vi "Testing Mode.vi"(8 "Filepath":path=path "D:/My Project/2019-2020/Magnetic Mareli UM/MM_UM/Project Setup/data/program seq/Program_280A.bin", 9 "FeedBack Channel":string[](array[string])=["fgdgfvcbc", "vnfhgjkn", "21354682"]) -> ()   [LabVIEW 2015]
uses:
  Control Button/Exit.ctl
  Control Button/Start.ctl
  Test  enqueue/AutoTest seq.ctl
  Control Button/Stop.ctl
  Control Button/Emergency.ctl
  Test  enqueue/Auot Test selection.ctl
  Galobal variable_TI.vi
  Project Setup/Globle Variable/GR_Servo.vi
  <vilib>/Utility/file.llb/Read Delimited Spreadsheet (string).vi
panel:
  out "Numeric":u32
  out "Error Message 2":string
  out "Sensor Setting Data":T1
  out "Sensor Data":T2
  out "Cllip-4 (AI12)":bool
  out "Cllip-3 (AI11)":bool
  out "Cllip-2(AI10)":bool
  out "Cllip-1 (AI9)":bool
  in  "Tracibility":bool=TRUE
  out "Home":bool
  out "Reset":bool
  out "Emergency":bool
  out "Start":bool
  out "Error   For Message":bool
  out "reset":bool
  out "D-enqueue":T3
  in  "Servo Fault Reset":bool
  out "Servo Fault":bool
  in  "Report":bool
  in  "Tab Control":enum32{"Test", "Report"}(tab)
  out "Error":bool
  out "User Name":string
  in  "Table Control":string[][](table)
  in  "OK Counter":string
  in  "NG Counter":string
  out "Running Model":string
  out "Date time":string
  out "TFT Barcode":string
  out "MIC Barcode":string
  out "2D Picture":picture
  out "Camera":bool
  out "Camera":bool
  out "Co-ordinate":string
  out "Test Name":string
  out "Error Message":string
  out "Boolean 2":bool
  in  "Report":i32(listbox)
  out "Key Pad AI1":bool
  out "Key Pad AI0":bool
  out "appended array":string[](array[string])
  in  "Sensor Feedback":T4(array[cluster])
  in  "Home Call":bool
  out "Start":bool
  in  "Cycle":i32
  in  "Slide Servo Home Call":bool
  in  "Emergency":T5
  in  "Stop":T6
  in  "Home Call":bool
  out "Current Date & Time":timestamp
  out "Cycle Time(Sec)":i32
  in  "Start":T7
  in  "Cycle Start Bit":bool
  in  "vi reference":refnum<vi>
  in  "Reset Ct.":bool
  out "error out":errorcluster
  in  "Tbl Refnum":refnum<vi>
  in  "Exit":T8
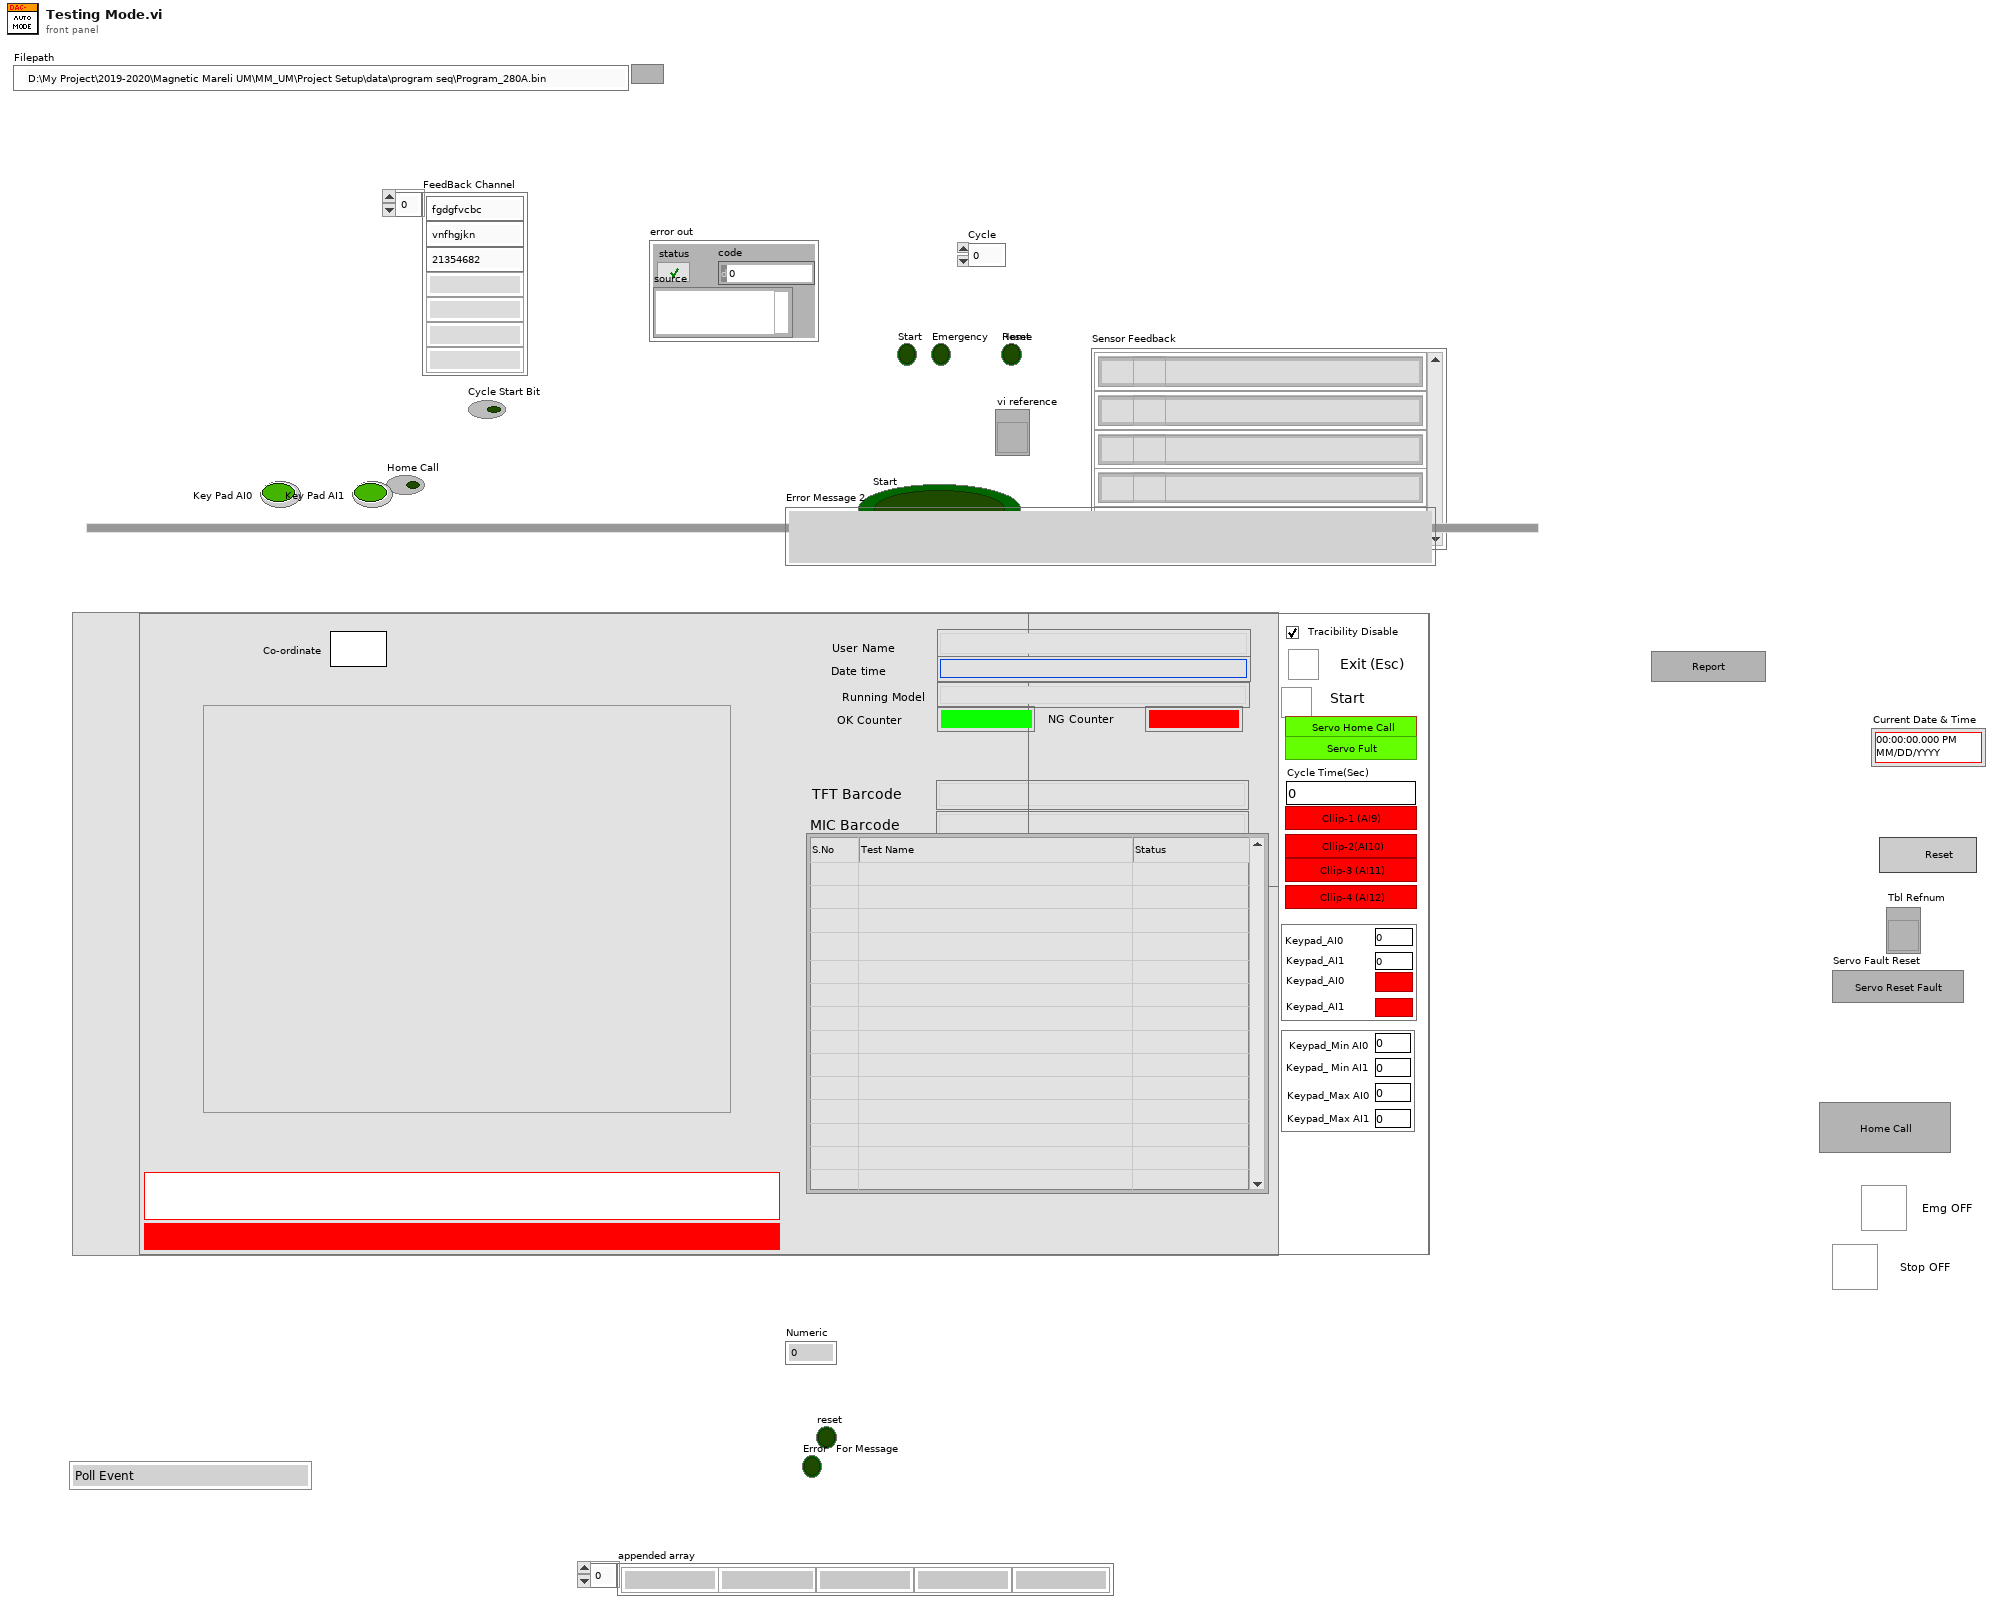
[diagram p1: front panel]
types:
  T1 = cluster{"Keypad_Max AI0":dbl, "Keypad_Min AI0":dbl, "Keypad_Max AI1":dbl, "Keypad_ Min AI1":dbl}
  T2 = cluster{"Keypad_AI0":dbl, "Keypad_AI1":dbl, "Keypad_AI0":bool, "Keypad_AI1":bool}
  T3 = typedef "AutoTest seq.ctl" = enum16{"Poll Event", "Part Clamp", "Program Seq", "Cylender Home", "Read Barcode", "Slide Servo send Cammand", "Slide Servo Home Call", "Camera Co-ordinate_1", "Camera Co-ordinate_2", "Result Save", "Error", "Exit"}
  T4 = cluster{"Sensor Name":string, "OK And NG":bool}[]
  T5 = typedef "Emergency.ctl" = bool
  T6 = typedef "Stop.ctl" = bool
  T7 = typedef "Start.ctl" = bool
  T8 = typedef "Exit.ctl" = bool
  T9 = cluster{"MIC ":refnum<visa-resource-name>, "baud rate MIC ":u32, "LCD ":refnum<visa-resource-name>, "baud rate_LCD":u32}
  T10 = typedef "Auot Test selection.ctl" = enum16{"Init", "Enqueue ", "Enqueue N", "Enqueue in stack", "Enqueue in stack N", "Dequeue", "Dequeue N", "Flush", "Release Queue"}
  T11 = cluster{"Item Name":string, "Item Status":bool, "Steps":cluster{"Channel Type":string, "Channels":string, "Wait/Poll (ms)":u32, "Parameter":u8, "STM-Speed":i32, "STM-Degree":u32, "Direction":u8}[]}[]
  T12 = enum16{"Part Clamp", "Part Unclamp", "Part Clamp Input Check", "Part Unclamp Input Check"}
  T13 = cluster{"No. Fail Coun t":string, "Rework Status Count 0\\1":string, "NA Count Max =3 ":string, "Testesd Count  0/1":string, "Error code":string}
  T14 = cluster{"Emergency_1":bool, "Reset_2":bool, "Air Pressure_4":bool, "Safety Sensor_5":bool, "Safety Sensor_6":bool, "Barcode Rev rs_24":bool, "Clamp fwd rs_21":bool, "Servo Fault":bool, "Home _3":bool}
  T15 = cluster{"IL Sensor1_Max AI0":dbl, "IL Sensor1_Min AI0":dbl, "IL Sensor1_Max AI1":dbl, "IL Sensor1_ Min AI1":dbl, "IL Sensor_Max (AI9)":dbl, "IL Sensor_Min  (AI9)":dbl, "IL Sensor_Max (AI10)":dbl, "IL Sensor_Min(AI10)":dbl, "IL Sensor_Max (AI11)":dbl, "IL Sensor_Min (AI11)":dbl, "IL Sensor_Max (AI12)":dbl, "IL Sensor_Min (AI12":dbl}
  T16 = cluster{"IL Sensor1_AI0":dbl, "IL Sensor1_AI1":dbl, "IL Sensor (AI6)":dbl, "IL Sensor  (AI7)":dbl, "IL Sensor (AI8)":dbl, "IL Sensor  (AI9)":dbl, "IL Sensor1_AI0":bool, "IL Sensor1_AI1":bool, "IL Sensor1_AI9":bool, "IL Sensor1_AI10":bool, "IL Sensor1_AI11":bool, "IL Sensor1_AI12":bool}
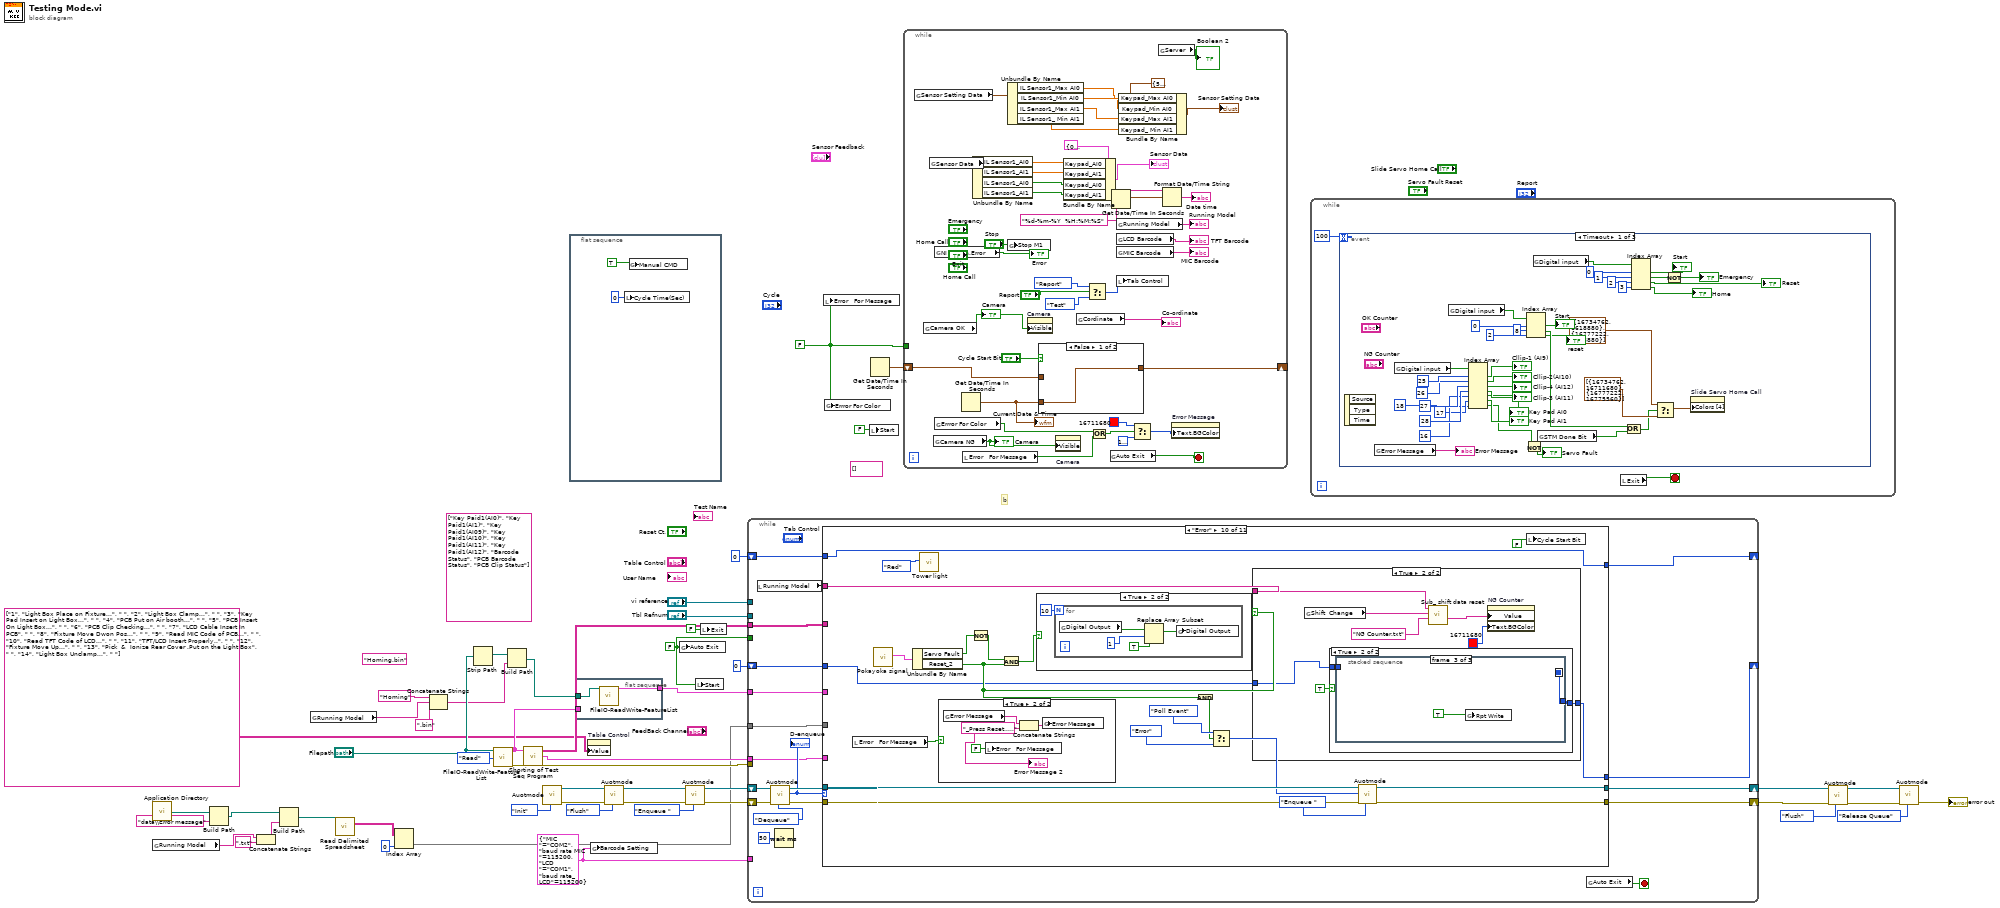
[diagram p0: block diagram]
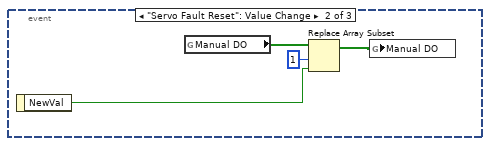
[diagram p2: hidden frame]
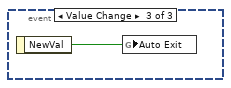
[diagram p3: hidden frame]
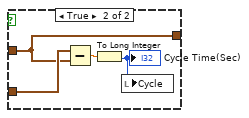
[diagram p4: hidden frame]
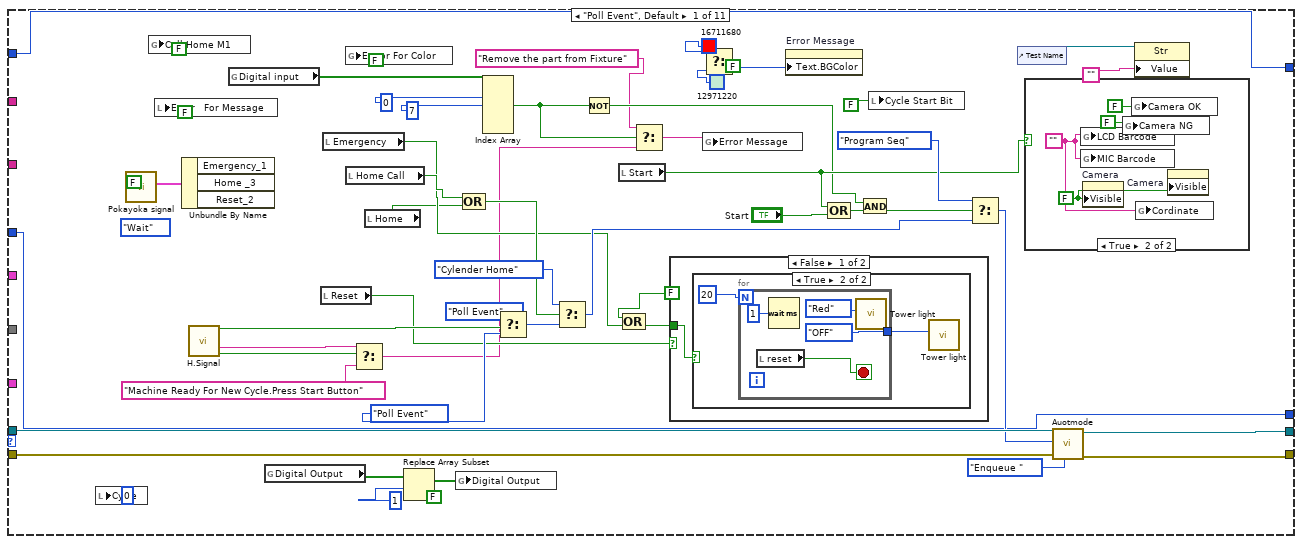
[diagram p5: hidden frame]
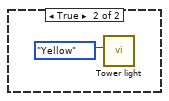
[diagram p8: hidden frame]
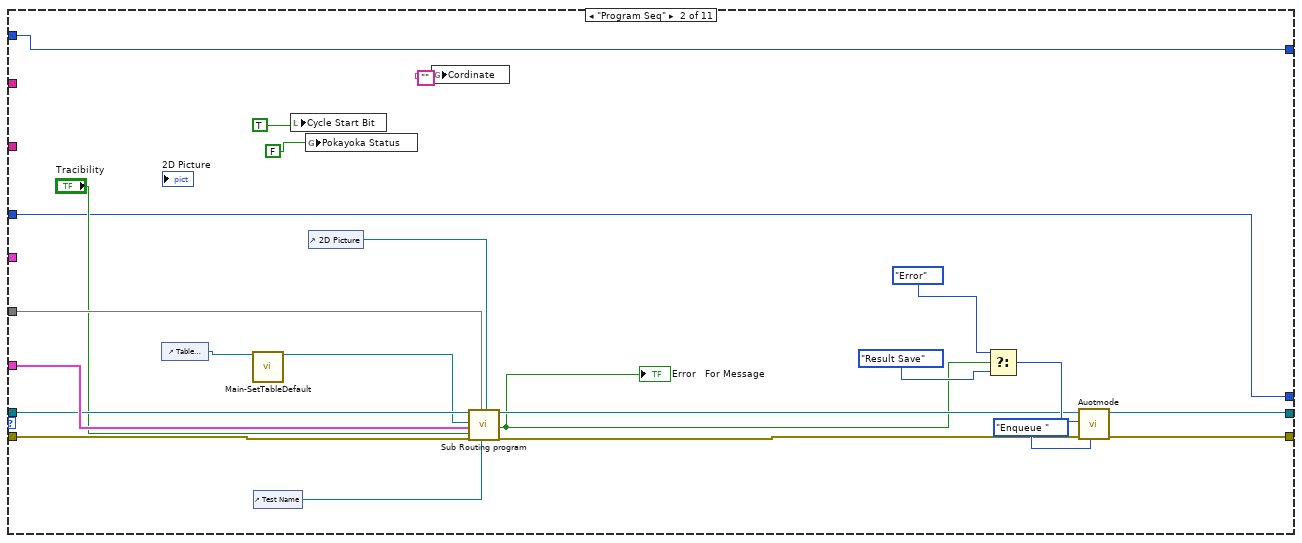
[diagram p9: hidden frame]
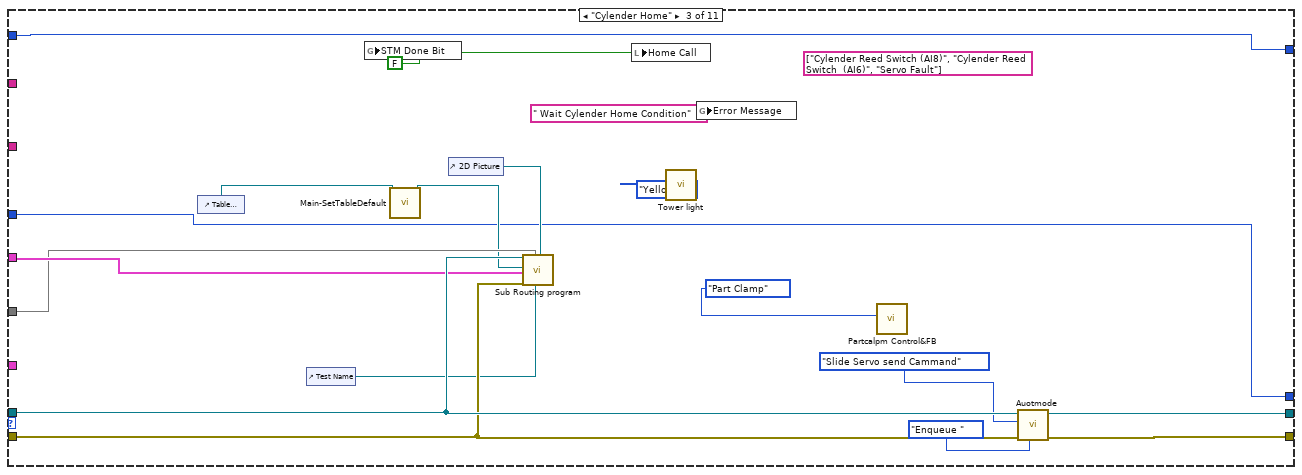
[diagram p10: hidden frame]
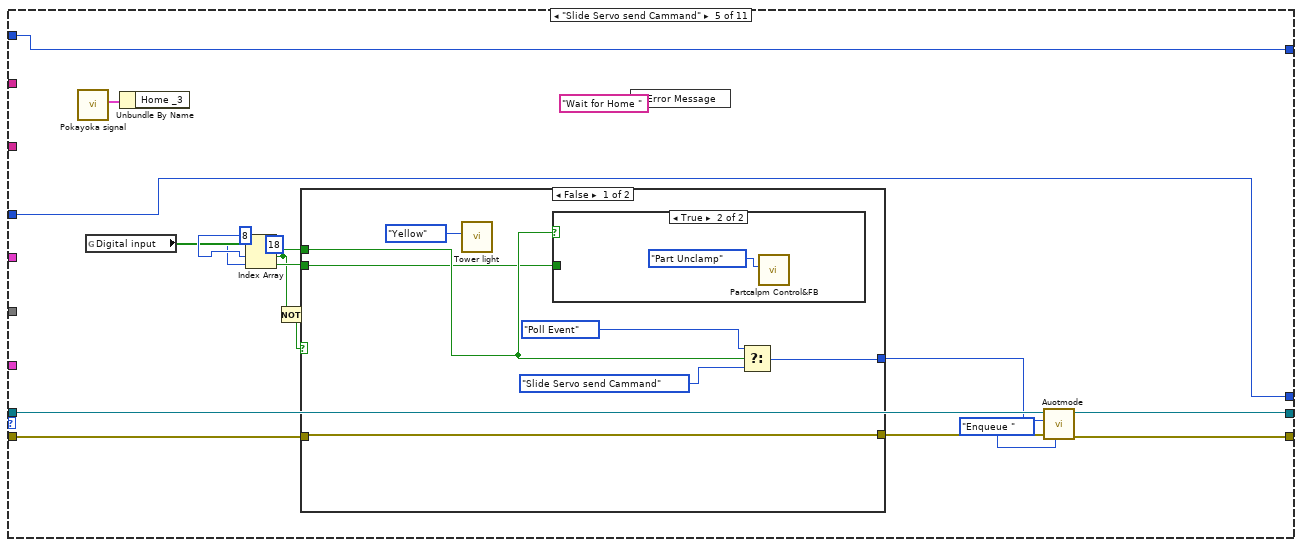
[diagram p12: hidden frame]
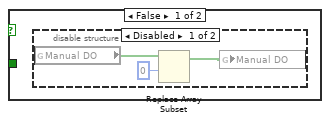
[diagram p13: hidden frame]
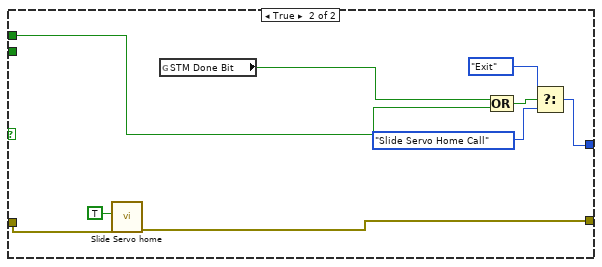
[diagram p15: hidden frame]
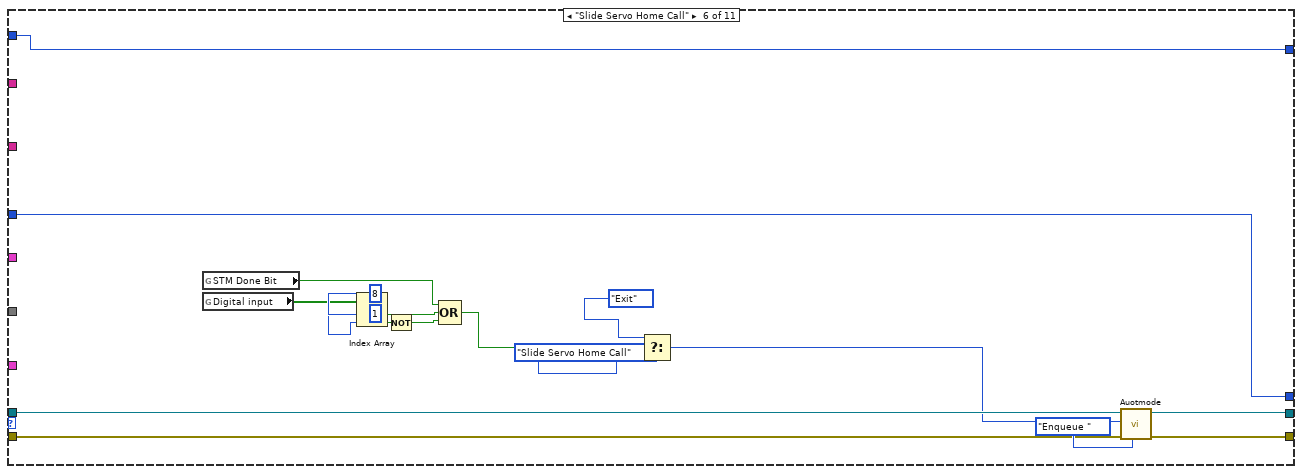
[diagram p16: hidden frame]
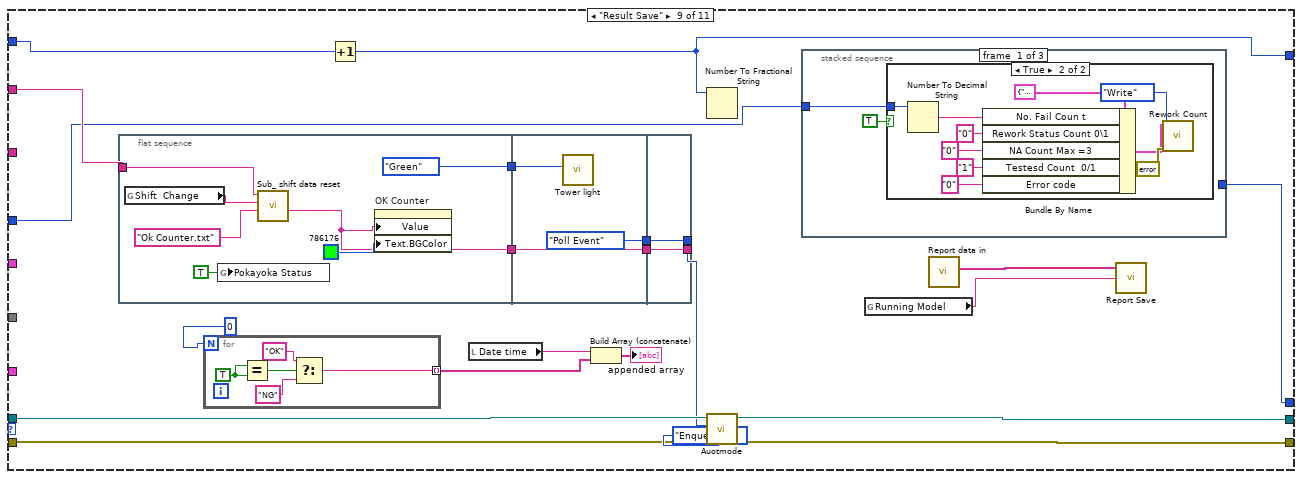
[diagram p19: hidden frame]
diagram:
  w20 = T9 {"MIC "="COM2", "baud rate MIC "=115200, "LCD "="COM1", "baud rate_LCD"=115200} ("Barcode Setting")
  (unwired) "Homing.bin" ("name or relative path")
  (unwired) string[] ["Key Paid1(AI0)", "Key Paid1(AI1)", "Key Paid1(AI09)", "Key Paid1(AI10)", "Key Paid1(AI11)", "Key Paid1(AI12)", "Barcode Status", "PCB Barcode Status", "PCB Clip Status"] ("Error Name")
  (unwired) string[] []
  w4 = FALSE ("Servo Stop")
  w27 = FALSE ("Auto Exit")
  # "b"
  n1 = call <vilib>:"Application Directory.vi"() -> ("Application Directory"=w14:path)
  n2 = global read "Galobal variable_TI.vi" "Running Model"() -> (w11:string)
  n3 = Build Path(base path=w14, name or relative path="data\\Error message") -> (appended path=w12:path)
  n4 = Concatenate Strings(w11, ".txt" ("string")) -> (w9:string)
  n5 = Build Path(base path=w12, name or relative path=w9) -> (appended path=w8:path)
  n6 = global read "Galobal variable_TI.vi" "Running Model"() -> (w18:string)
  n7 = call-poly <vilib>:"Read Delimited Spreadsheet.vi"("file path (dialog if empty)"=w8) -> ("all rows"=w7:string[][])  [unwired: 9 in, 5 out]
  n8 = Index Array(array=w7, index (col)=0 ("disabled index (col)")) -> (element=w5:string[])  [unwired: 1 in]
  n9 = Concatenate Strings("Homing" ("string"), w18, ".bin" ("string")) -> (w16:string)
  n10 = Strip Path(path="Filepath") -> (stripped path=w24:path)  [unwired: 1 out]
  n11 = call "FileIO-ReadWrite-FeatureList.vi"("Filepath"="Filepath", "Read/Write"=enum16{"Read", "Write"}."Read") -> ("Feature List (Out)"=w22:T11, "Error Out"=w32:errorcluster)  [unwired: 12 in]
  n12 = Build Path(base path=w24, name or relative path=w16) -> (appended path=w23:path)
  n13 = call "Shorting of Test Seq Program.vi"("Feature List (Out)"=w22) -> ("Feature Step Enable"=w28:T11, "Feature Name"=w3:string[][])  [unwired: 3 in]
  n14 = call "Auotmode.vi"("Enum Selection"=Auot_Test_selection."Init") -> ("error out"=w44:errorcluster, "queue Out"=w42:refnum<queue>)  [unwired: 7 in, 1 out]
  n15 = flat-sequence {
    frame #0 {
      n16 = local write "Cycle Time(Sec)"(0 ("Cycle Time(Sec)")) -> ()
      n17 = global write "Galobal variable_TI.vi" "Manual CMD"(TRUE ("Manual CMD")) -> ()
    }
  }
  n18 = flat-sequence {
    tunnel: w23 -> [w54]
    tunnel: w22 -> [_]
    tunnel: [w53] -> w21
    frame #0 {
      n19 = call "FileIO-ReadWrite-FeatureList.vi"("Filepath"=w54) -> ("Feature List (Out)"=w53:T11)  [unwired: 13 in, 1 out]
    }
  }
  n20 = property on="Table Control" class="Tbl (strict)"("Value"=string[][] [["1", "Light Box Place on Fixture...", " "], ["2", "Light Box Clamp...", " "], ["3", "Key Pad Insert on Light Box...", " "], ["4", "PCB Put on Air booth...", " "], ["5", "PCB Insert On Light Box...", " "], ["6", "PCB Clip Checking...", " "], ["7", "LCD Cable Insert In PCB", " "], ["8", "Fixture Move Dwon Pos...", " "], ["9", "Read MIC Code of PCB...", " "], ["10", "Read TFT Code of LCD...", " "], ["11", "TFT/LCD Insert Properly..", " "], ["12", "Fixture Move Up...", " "], ["13", "Pick  &  Ionize Rear Cover .Put on the Light Box", " "], ["14", "Light Box Unclamp...", " "]] ("Table Control 2")) -> ()  [unwired: 2 in, 2 out]
  n21 = global write "Galobal variable_TI.vi" "Barcode Setting"(w20) -> ()
  n22 = call "Auotmode.vi"("Enum Selection"=Auot_Test_selection."Flush", "Error In"=w44, "queue in"=w42) -> ("error out"=w43:errorcluster, "queue Out"=w41:refnum<queue>)  [unwired: 5 in, 1 out]
  n23 = global write "Galobal variable_TI.vi" "Auto Exit"(w27) -> ()
  n24 = call "Auotmode.vi"("Enum Selection"=Auot_Test_selection."Enqueue ", "Error In"=w43, "queue in"=w41) -> ("error out"=w48:errorcluster, "queue Out"=w30:refnum<queue>)  [unwired: 5 in, 1 out]
  n25 = local write "Start"(w27) -> ()
  n26 = local write "Exit"(T8 FALSE ("Exit")) -> ()
  n27 = while {
    tunnel: "vi reference" -> [_]
    tunnel: "Tbl Refnum" -> [_]
    tunnel: w28 -> [w66]
    tunnel: w32 -> [_]
    tunnel: w5 -> [w67]
    shift-right: [w70] -> w35
    shift-left: w30 -> [w63]
    shift-right: [w62] -> w29
    shift-left: w48 -> [w72]
    tunnel: w27 -> [_]
    tunnel: w3 -> [w61]
    tunnel: w21 -> [w59]
    tunnel: w20 -> [_]
    shift-right: [w57] -> _
    shift-left: u32 0 ("milliseconds to wait") -> [w58]
    shift-right: [w55] -> _
    shift-left: u32 0 ("milliseconds to wait") -> [w56]
    stop <- w65 stop-if-true
    n28 = local read "Running Model"() -> (w60:string)
    n29 = call "Auotmode.vi"("Enum Selection"=Auot_Test_selection."Dequeue", "Error In"=w72, "queue in"=w63) -> ("error out"=w69:errorcluster, "D-enqueue"=w68:T3, "queue Out"=w71:refnum<queue>)  [unwired: 5 in]
    "D-enqueue" <- w68
    n30 = Wait (ms)(milliseconds to wait=u32 50) -> ()  [unwired: 1 out]
    n31 = case shown="\"Error\"" w68 {
      tunnel: w71 -> [w126 w151 w175 w183 w195 w235 w242 w246 w266 w319 w365]
      tunnel: [w124 w157 w178 w183 w199 w236 w242 w246 w264 w318 w366] -> w70
      tunnel: w69 -> [w125 w153 w174 w182 w197 w234 w241 w245 w265 w317 w367]
      tunnel: [w123 w156 w177 w182 w198 w237 w241 w245 w263 w316 w367] -> w62
      tunnel: w66 -> [_ w154 _ _ _ _ _ _ _ _ _]
      tunnel: w67 -> [_ w155 w172 _ _ _ _ _ _ _ _]
      tunnel: w61 -> [_ _ _ _ _ _ _ _ _ _ _]
      tunnel: w60 -> [_ _ _ _ _ _ _ _ w262 w310 _]
      tunnel: w59 -> [_ _ w173 _ _ _ _ _ _ _ _]
      tunnel: w58 -> [w87 w142 w163 w181 w185 w222 w240 w244 w251 w302 w358]
      tunnel: [w87 w142 w163 w181 w185 w222 w240 w244 w250 w302 w358] -> w57
      tunnel: w56 -> [w80 w139 w162 w180 w184 w221 w239 w243 w248 w301 w357]
      tunnel: [w80 w139 w162 w180 w184 w221 w239 w243 w247 w300 w357] -> w55
      frame "Poll Event", Default {
        (unwired) enum16{"Wait", "Ionizer On", "Ionizer off"}."Wait" ("Enum")
        (unwired) FALSE ("Ionizer cnf")
        n32 = local write "Cycle"(0 ("Cycle")) -> ()
        n33 = call "Pokayoka signal.vi"() -> ("output cluster"=w105:T14)  [unwired: 10 in, 1 out]
        n34 = global write "Galobal variable_TI.vi" "Call Home M1"(FALSE ("Call Home M1")) -> ()
        n35 = local write "Error   For Message"(FALSE ("Error   For Message")) -> ()
        n36 = Unbundle By Name(w105) -> ()  [unwired: 3 out]
        n37 = call "H.Signal.vi"() -> ("Slide servo home RS"=w111:bool, "Error Message"=w112:string, "Bool_H Sig"=w99:bool)  [unwired: 10 in, 3 out]
        n38 = global read "Galobal variable_TI.vi" "Digital input"() -> (w121:bool[])
        n39 = global read "Galobal variable_TI.vi" "Digital Output"() -> (w96:bool[])
        n40 = local read "Reset"() -> (w83:bool)
        n41 = local read "Emergency"() -> (w85:bool)
        n42 = global write "Galobal variable_TI.vi" "Errror For Color"(FALSE ("Errror For Color")) -> ()
        n43 = local read "Home Call"() -> (w97:bool)
        n44 = Select(t=w112, s=w99, f="Machine Ready For New Cycle.Press Start Button") -> (s? t:f=w74:string)
        n45 = local read "Home"() -> (w84:bool)
        n46 = Replace Array Subset(array=w96, new element=FALSE ("new element/subarray"), index=1) -> (w95:bool[])
        n47 = global write "Galobal variable_TI.vi" "Digital Output"(w95) -> ()
        n48 = Compound Arithmetic op=OR(w97, w84) -> (w118:bool)
        n49 = Index Array(array=w121, index #1=0 ("index"), index #2=7 ("index")) -> (element #2=w75:bool)  [unwired: 3 in, 4 out]
        n50 = Select(t=AutoTest_seq."Poll Event" ("Enqueue"), s=w111, f=AutoTest_seq."Poll Event") -> (s? t:f=w116:T3)
        n51 = Select(t=AutoTest_seq."Cylender Home" ("Enqueue"), s=w118, f=w116) -> (s? t:f=w104:T3)
        n52 = Not(x=w75) -> (.not. x?=w78:bool)
        n53 = local read "Start"() -> (w86:bool)
        n54 = Compound Arithmetic op=OR(FALSE ("value"), w85) -> (w100:bool)
        n55 = Select(t="Remove the part from Fixture", s=w75, f=w74) -> (s? t:f=w77:string)
        n56 = case shown="False" w83 {
          tunnel: w100 -> [w131 _]
          frame False {
            n57 = case shown="True" w131 {
              frame False {
              }
              frame True {
                n58 = for {
                  N: 20 -> [_]
                  tunnel: [enum16{"Green", "Red", "Yellow", "OFF"}."OFF" ("Enum")] -> w132
                  stop <- w134 stop-if-true
                  n59 = local read "reset"() -> (w134:bool)
                  n60 = Wait (ms)(milliseconds to wait=u32 1) -> ()  [unwired: 1 out]
                  n61 = call "Tower light.vi"("Enum"=enum16{"Green", "Red", "Yellow"}."Red") -> ()  [unwired: 11 in]
                }
                n62 = call "Tower light.vi"("Enum"=w132) -> ()  [unwired: 11 in]
              }
            }
          }
          frame True {
            n63 = call "Tower light.vi"("Enum"=enum16{"Green", "Red", "Yellow"}."Yellow") -> ()  [unwired: 11 in]
          }
        }
        n64 = global write "GR_Servo.vi" "Error Message"(w77) -> ()
        n65 = Select(t=u32 16711680, s=FALSE, f=u32 12971220) -> (s? t:f=w88:u32)
        n66 = property on="Error Message" class="Str"("Text.BGColor"=w88) -> ()  [unwired: 2 in, 2 out]
        n67 = Compound Arithmetic op=OR(w86, "Start") -> (w109:T7)
        n68 = And(x=w78, y=w109) -> (x .and. y?=w79:T7)
        n69 = local write "Cycle Start Bit"(FALSE ("Cycle Start Bit")) -> ()
        n70 = Select(t=AutoTest_seq."Program Seq" ("Enqueue"), s=w79, f=w104) -> (s? t:f=w103:T3)
        n71 = control-ref of="Test Name"() -> (w102:refnum<vi>)
        n72 = case shown="True" w86 {
          frame False {
          }
          frame True {
            w130 = FALSE ("Visible")
            w127 = ""
            n73 = global write "Galobal variable_TI.vi" "LCD Barcode"(w127) -> ()
            n74 = global write "Galobal variable_TI.vi" "MIC Barcode"(w127) -> ()
            n75 = property on="Camera" class="Bool (strict)"("Visible"=w130) -> ()  [unwired: 2 in, 2 out]
            n76 = global write "Galobal variable_TI.vi" "Camera NG"(FALSE ("Camera NG")) -> ()
            n77 = global write "Galobal variable_TI.vi" "Camera OK"(FALSE ("Camera OK")) -> ()
            n78 = global write "Galobal variable_TI.vi" "Cordinate"(w127) -> ()
            n79 = property on="Camera" class="Bool (strict)"("Visible"=w130) -> ()  [unwired: 2 in, 2 out]
          }
        }
        n80 = call "Auotmode.vi"("Enum Selection"=Auot_Test_selection."Enqueue ", "Error In"=w125, "Enqueue"=w103, "queue in"=w126) -> ("error out"=w123:errorcluster, "queue Out"=w124:refnum<queue>)  [unwired: 4 in, 1 out]
        n81 = property class="Str"(reference=w102, "Value"="") -> ()  [unwired: 1 in, 2 out]
      }
      frame "Program Seq" {
        n82 = control-ref of="Table Control"() -> (w147:refnum<vi>)
        n83 = call "Main-SetTableDefault.vi"("Table (In)"=w147) -> ("Table (Out)"=w146:refnum<vi>)  [unwired: 13 in, 1 out]
        n84 = control-ref of="Test Name"() -> (w149:refnum<vi>)
        n85 = local write "Cycle Start Bit"(TRUE ("Cycle Start Bit")) -> ()
        n86 = global write "Galobal variable_TI.vi" "Pokayoka Status"(FALSE ("Pokayoka Status")) -> ()
        n87 = control-ref of="2D Picture"() -> (w148:refnum<vi>)
        n88 = global write "Galobal variable_TI.vi" "Cordinate"("") -> ()
        n89 = call "Sub Routing program.vi"("queue Out in"=w151, "Table"=w146, "Feature Step Enable"=w154, "error in (no error)"=w153, "Tracibility"="Tracibility", "FeedBack Channel"=w155, "Test Name"=w149, "Image"=w148) -> ("Queue out"=w150:refnum<queue>, "Error"=w143:bool, "error out"=w152:errorcluster)  [unwired: 8 in, 1 out]
        "Error   For Message" <- w143
        n90 = Select(t=AutoTest_seq."Error" ("Enqueue"), s=w143, f=AutoTest_seq."Result Save" ("Enqueue")) -> (s? t:f=w158:T3)
        n91 = call "Auotmode.vi"("Enum Selection"=Auot_Test_selection."Enqueue ", "Error In"=w152, "Enqueue"=w158, "queue in"=w150) -> ("error out"=w156:errorcluster, "queue Out"=w157:refnum<queue>)  [unwired: 4 in, 1 out]
      }
      frame "Cylender Home" {
        (unwired) string[] ["Cylender Reed Switch (AI8)", "Cylender Reed Switch  (AI6)", "Servo Fault"]
        w176 = FALSE ("STM Done Bit")
        n92 = control-ref of="Table Control"() -> (w168:refnum<vi>)
        n93 = control-ref of="Test Name"() -> (w171:refnum<vi>)
        n94 = global write "Galobal variable_TI.vi" "STM Done Bit"(w176) -> ()
        n95 = call "Main-SetTableDefault.vi"("Table (In)"=w168) -> ("Table (Out)"=w167:refnum<vi>)  [unwired: 13 in, 1 out]
        n96 = control-ref of="2D Picture"() -> (w170:refnum<vi>)
        n97 = call "Sub Routing program.vi"("queue Out in"=w175, "Table"=w167, "Feature Step Enable"=w173, "error in (no error)"=w174, "FeedBack Channel"=w172, "Test Name"=w171, "Image"=w170) -> ()  [unwired: 9 in, 4 out]
        n98 = local write "Home Call"(w176) -> ()
        n99 = call "Tower light.vi"("Enum"=enum16{"Green", "Red", "Yellow"}."Yellow") -> ()  [unwired: 11 in]
        n100 = global write "GR_Servo.vi" "Error Message"(" Wait Cylender Home Condition") -> ()
        n101 = call "Partcalpm Control&FB.vi"("Enum"=T12."Part Clamp") -> ()  [unwired: 9 in, 2 out]
        n102 = call "Auotmode.vi"("Enum Selection"=Auot_Test_selection."Enqueue ", "Error In"=w174, "Enqueue"=AutoTest_seq."Slide Servo send Cammand", "queue in"=w175) -> ("error out"=w177:errorcluster, "queue Out"=w178:refnum<queue>)  [unwired: 4 in, 1 out]
      }
      frame "Read Barcode" {
      }
      frame "Slide Servo send Cammand" {
        n103 = call "Pokayoka signal.vi"() -> ("output cluster"=w193:T14)  [unwired: 10 in, 1 out]
        n104 = global read "Galobal variable_TI.vi" "Digital input"() -> (w190:bool[])
        n105 = Unbundle By Name(w193) -> ()  [unwired: 1 out]
        n106 = Index Array(array=w190, index #1=8 ("index"), index #2=18 ("index")) -> (element #1=w187:bool, element #2=w188:bool)
        n107 = Not(x=w187) -> (.not. x?=w186:bool)
        n108 = case shown="False" w186 {
          tunnel: w197 -> [w207 w220]
          tunnel: [w207 w219] -> w196
          tunnel: [w203 w214] -> w194
          tunnel: w187 -> [w202 w212]
          tunnel: w188 -> [w201 _]
          frame False {
            n109 = call "Tower light.vi"("Enum"=enum16{"Green", "Red", "Yellow"}."Yellow") -> ()  [unwired: 11 in]
            n110 = case shown="True" w202 {
              tunnel: w201 -> [_ _]
              frame False {
                n111 = disable-structure shown="Disabled" {
                  frame Disabled {
                    n112 = global read "Galobal variable_TI.vi" "Manual DO"() -> (w210:bool[])
                    n113 = Replace Array Subset(array=w210, index=0) -> (w209:bool[])  [unwired: 1 in]
                    n114 = global write "Galobal variable_TI.vi" "Manual DO"(w209) -> ()
                  }
                  frame Enabled {
                  }
                }
              }
              frame True {
                n115 = call "Partcalpm Control&FB.vi"("Enum"=T12."Part Unclamp") -> ()  [unwired: 9 in, 2 out]
              }
            }
            n116 = Select(t=AutoTest_seq."Poll Event" ("Enqueue"), s=w202, f=AutoTest_seq."Slide Servo send Cammand" ("Enqueue")) -> (s? t:f=w203:T3)
          }
          frame True {
            n117 = call "Slide Servo home.vi"("error in"=w220, "NewVal"=TRUE) -> ("error out"=w219:errorcluster)  [unwired: 9 in]
            n118 = global read "Galobal variable_TI.vi" "STM Done Bit"() -> (w217:bool)
            n119 = Compound Arithmetic op=OR(w217, w212) -> (w213:bool)
            n120 = Select(t=AutoTest_seq."Exit" ("Enqueue"), s=w213, f=AutoTest_seq."Slide Servo Home Call" ("Enqueue")) -> (s? t:f=w214:T3)
          }
        }
        n121 = global write "GR_Servo.vi" "Error Message"("Wait for Home ") -> ()
        n122 = call "Auotmode.vi"("Enum Selection"=Auot_Test_selection."Enqueue ", "Error In"=w196, "Enqueue"=w194, "queue in"=w195) -> ("error out"=w198:errorcluster, "queue Out"=w199:refnum<queue>)  [unwired: 4 in, 1 out]
      }
      frame "Slide Servo Home Call" {
        n123 = global read "Galobal variable_TI.vi" "STM Done Bit"() -> (w228:bool)
        n124 = global read "Galobal variable_TI.vi" "Digital input"() -> (w226:bool[])
        n125 = Index Array(array=w226, index #1=8 ("index"), index #2=1 ("index")) -> (element #1=w227:bool, element #2=w224:bool)
        n126 = Not(x=w224) -> (.not. x?=w223:bool)
        n127 = Compound Arithmetic op=OR(w228, w227, w223) -> (w230:bool)
        n128 = Select(t=AutoTest_seq."Exit" ("Enqueue"), s=w230, f=AutoTest_seq."Slide Servo Home Call" ("Enqueue")) -> (s? t:f=w233:T3)
        n129 = call "Auotmode.vi"("Enum Selection"=Auot_Test_selection."Enqueue ", "Error In"=w234, "Enqueue"=w233, "queue in"=w235) -> ("error out"=w237:errorcluster, "queue Out"=w236:refnum<queue>)  [unwired: 4 in, 1 out]
      }
      frame "Camera Co-ordinate_1" {
      }
      frame "Camera Co-ordinate_2" {
      }
      frame "Result Save" {
        n130 = flat-sequence {
          tunnel: w262 -> [w292]
          tunnel: [enum16{"Green", "Red", "Yellow"}."Green" ("Enum")] -> w261
          tunnel: [w289] -> w253
          tunnel: w261 -> [w297]
          tunnel: [AutoTest_seq."Poll Event" ("Enqueue")] -> w259
          tunnel: [w295] -> w254
          tunnel: w253 -> [w295]
          tunnel: [w299] -> w260
          tunnel: w259 -> [w299]
          tunnel: [w298] -> _
          tunnel: w254 -> [w298]
          frame #0 {
            n131 = global read "Galobal variable_TI.vi" "Shift  Change"() -> (w288:string)
            n132 = global write "Galobal variable_TI.vi" "Pokayoka Status"(TRUE ("Pokayoka Status")) -> ()
            n133 = call "Sub_ shift data reset.vi"("Serial no"="Ok Counter.txt" ("File Name"), "Shift"=w288, "Model"=w292) -> ("Serial no"=w289:string)  [unwired: 6 in, 1 out]
            n134 = property on="OK Counter" class="Str"("Value"=w289, "Text.BGColor"=u32 786176 ("Color Box")) -> ()  [unwired: 2 in, 2 out]
          }
          frame #1 {
            n135 = call "Tower light.vi"("Enum"=w297) -> ()  [unwired: 11 in]
          }
          frame #2 {
          }
        }
        n136 = for {
          N: 0 -> [_]
          tunnel: [w284] -> w257 mode=indexing
          w283 = TRUE ("y")
          n137 = Equal?(x=w283, y=w283) -> (x = y?=w287:bool)
          n138 = Select(t="OK", s=w287, f="NG") -> (s? t:f=w284:string)
        }
        n139 = Increment(x=w251) -> (x+1=w250:u32)
        n140 = local read "Date time"() -> (w258:string)
        n141 = Build Array (concatenate)(w258, w257) -> (→"appended array":string[])
        n142 = Number To Fractional String(number=w250) -> ()  [unwired: 3 in, 1 out]
        n143 = call "Auotmode.vi"("Enum Selection"=Auot_Test_selection."Enqueue ", "Error In"=w265, "Enqueue"=w260, "queue in"=w266) -> ("error out"=w263:errorcluster, "queue Out"=w264:refnum<queue>)  [unwired: 4 in, 1 out]
        n144 = stacked-sequence {
          tunnel: w248 -> [w269 _ _]
          tunnel: [_ u32 0 ("milliseconds to wait") _] -> w247
          frame #0 {
            n145 = case shown="True" TRUE {
              tunnel: w269 -> [_ w273]
              frame False {
              }
              frame True {
                n146 = Number To Decimal String(number=w273) -> (decimal integer string=w274:string)  [unwired: 1 in]
                n147 = Bundle By Name(cluster=T13 {"No. Fail Coun t"="", "Rework Status Count 0\\1"="", "NA Count Max =3 "="", "Testesd Count  0/1"="", "Error code"=""} ("Count For Rework"), "No. Fail Coun t"=w274, "Rework Status Count 0\\1"="0" ("Rework Status Count 0\\1"), "NA Count Max =3"="0", "Testesd Count  0/1"="1", "Error code"="0") -> (w271:T13)
                n148 = call "Rework Count.vi"("error in"=errorcluster {"status"=FALSE, "code"=0, "source"=""}, "Read /Write"=enum16{"Write", "Read"}."Write", "Count For Rework"=w271) -> ()  [unwired: 7 in, 2 out]
              }
            }
          }
          frame #1 {
            n149 = Wait (ms)(milliseconds to wait=u32 200) -> ()  [unwired: 1 out]
          }
          frame #2 {
            n150 = global write "Galobal variable_TI.vi" "Rpt Write"(TRUE) -> ()
          }
        }
        n151 = global read "Galobal variable_TI.vi" "Running Model"() -> (w252:string)
        n152 = call "Report data in.vi"() -> ("Report data"=w249:string[])  [unwired: 11 in]
        n153 = call "Report Save.vi"("Model No."=w252, "Report data"=w249) -> ()  [unwired: 4 in]
      }
      frame "Error" {
        n154 = local read "Error   For Message"() -> (w304:bool)
        n155 = call "Pokayoka signal.vi"() -> ("output cluster"=w314:T14)  [unwired: 10 in, 1 out]
        n156 = Unbundle By Name(w314) -> ("Servo Fault"=w307:bool, "Reset_2"=w308:bool)
        n157 = call "Tower light.vi"("Enum"=enum16{"Green", "Red", "Yellow"}."Red") -> ()  [unwired: 11 in]
        n158 = case shown="True" w304 {
          frame False {
          }
          frame True {
            n159 = global read "GR_Servo.vi" "Error Message"() -> (w324:string)
            "Error Message 2" <- w324
            n160 = local write "Error   For Message"(FALSE ("Error   For Message")) -> ()
            n161 = Concatenate Strings(w324, "_Press Reset....." ("string")) -> (w322:string)
            n162 = global write "GR_Servo.vi" "Error Message"(w322) -> ()
          }
        }
        n163 = Not(x=w307) -> (.not. x?=w305:bool)
        n164 = And(x=w305, y=w308) -> (x .and. y?=w306:bool)
        n165 = case shown="True" w306 {
          frame False {
          }
          frame True {
            n166 = for {
              N: 10 -> [_]
              n167 = global read "Galobal variable_TI.vi" "Digital Output"() -> (w329:bool[])
              n168 = Replace Array Subset(array=w329, new element=TRUE ("new element/subarray"), index=1) -> (w328:bool[])
              n169 = global write "Galobal variable_TI.vi" "Digital Output"(w328) -> ()
            }
          }
        }
        n170 = Compound Arithmetic op=AND(w308) -> (w303:bool)
        n171 = Select(t=AutoTest_seq."Poll Event" ("Enqueue"), s=w303, f=AutoTest_seq."Error" ("Enqueue")) -> (s? t:f=w311:T3)
        n172 = case shown="True" w308 {
          tunnel: w310 -> [_ w336]
          tunnel: w301 -> [w330 w335]
          tunnel: [w330 w334] -> w300
          frame False {
          }
          frame True {
            n173 = global read "Galobal variable_TI.vi" "Shift  Change"() -> (w332:string)
            n174 = case shown="True" TRUE {
              tunnel: w335 -> [w339 w341]
              tunnel: [w339 w340] -> w334
              frame False {
              }
              frame True {
                n175 = stacked-sequence {
                  seq-local: [w342 _ _] -> [_ w353 w355]
                  tunnel: w341 -> [w350 _ _]
                  tunnel: [_ _ w355] -> w340
                  frame #0 {
                    n176 = local read "Error Message 2"() -> (w343:string)
                    n177 = Increment(x=w350) -> (x+1=w342:u32)
                    n178 = Number To Decimal String(number=w342) -> (decimal integer string=w346:string)  [unwired: 1 in]
                    n179 = Bundle By Name(cluster=T13 {"No. Fail Coun t"="", "Rework Status Count 0\\1"="", "NA Count Max =3 "="", "Testesd Count  0/1"="", "Error code"=""} ("Count For Rework"), "No. Fail Coun t"=w346, "Rework Status Count 0\\1"="1" ("Rework Status Count 0\\1"), "NA Count Max =3"="1", "Testesd Count  0/1"="0", "Error code"=w343) -> (w344:T13)
                    n180 = call "Rework Count.vi"("error in"=errorcluster {"status"=FALSE, "code"=0, "source"=""}, "Read /Write"=enum16{"Write", "Read"}."Write", "Count For Rework"=w344) -> ()  [unwired: 7 in, 2 out]
                  }
                  frame #1 {
                    n181 = Wait (ms)(milliseconds to wait=u32 200) -> ()  [unwired: 1 out]
                    "Numeric" <- w353
                  }
                  frame #2 {
                    n182 = global write "Galobal variable_TI.vi" "Rpt Write"(TRUE) -> ()
                  }
                }
              }
            }
            n183 = call "Sub_ shift data reset.vi"("Serial no"="NG Counter.txt" ("File Name"), "Shift"=w332, "Model"=w336) -> ("Serial no"=w333:string)  [unwired: 6 in, 1 out]
            n184 = property on="NG Counter" class="Str"("Value"=w333, "Text.BGColor"=u32 16711680 ("Color Box")) -> ()  [unwired: 2 in, 2 out]
          }
        }
        n185 = call "Auotmode.vi"("Enum Selection"=Auot_Test_selection."Enqueue ", "Error In"=w317, "Enqueue"=w311, "queue in"=w319) -> ("error out"=w316:errorcluster, "queue Out"=w318:refnum<queue>)  [unwired: 4 in, 1 out]
        n186 = local write "Cycle Start Bit"(FALSE ("Cycle Start Bit")) -> ()
      }
      frame "Exit" {
        n187 = global read "Galobal variable_TI.vi" "Digital input"() -> (w362:bool[])
        n188 = Index Array(array=w362, index=8) -> (element=w359:bool)
        n189 = case shown="False" w359 {
          tunnel: [w369 w382] -> w364
          tunnel: ["Waitin servo home posi......" ("Error Message") "Home  Button Pressed" ("Error Message")] -> w360
          frame False {
            n190 = call "Pokayoka signal.vi"() -> ("output cluster"=w372:T14)  [unwired: 10 in, 1 out]
            n191 = Unbundle By Name(w372) -> ("Reset_2"=w371:bool)
            n192 = Select(t=AutoTest_seq."Poll Event" ("Enqueue"), s=w371, f=AutoTest_seq."Exit" ("Enqueue")) -> (s? t:f=w369:T3)
          }
          frame True {
            n193 = global read "Galobal variable_TI.vi" "Digital input"() -> (w388:bool[])
            n194 = global read "Galobal variable_TI.vi" "Manual DO"() -> (w380:bool[])
            n195 = Index Array(array=w388, index #1=22 ("index"), index #2=1 ("index")) -> (element #1=w377:bool, element #2=w376:bool)
            n196 = Replace Array Subset(array=w380, new element #1=FALSE ("new element/subarray"), index #1=4 ("index"), new element #2=TRUE ("new element/subarray"), index #2=5 ("index"), new element #3=FALSE ("new element/subarray"), index #3=10 ("index")) -> (w379:bool[])
            n197 = local write "Start"(T7 FALSE ("Start")) -> ()
            n198 = And(x=w377, y=w376) -> (x .and. y?=w375:bool)
            n199 = flat-sequence {
              tunnel: w379 -> [_]
              frame #0 {
                n200 = Wait (ms)(milliseconds to wait=u32 100) -> ()  [unwired: 1 out]
              }
            }
            n201 = global write "Galobal variable_TI.vi" "Manual DO"(w379) -> ()
            n202 = Select(t=AutoTest_seq."Poll Event" ("Enqueue"), s=w375, f=AutoTest_seq."Exit" ("Enqueue")) -> (s? t:f=w383:T3)
            n203 = case shown="True" w377 {
              tunnel: w379 -> [_ _]
              tunnel: [w395 w396] -> w382
              tunnel: w383 -> [w395 w396]
              frame False {
              }
              frame True {
                n204 = call "Tower light.vi"("Enum"=enum16{"Green", "Red", "Yellow"}."Green") -> ()  [unwired: 11 in]
              }
            }
          }
        }
        n205 = call "Auotmode.vi"("Enum Selection"=Auot_Test_selection."Enqueue ", "Enqueue"=w364, "queue in"=w365) -> ("queue Out"=w366:refnum<queue>)  [unwired: 5 in, 2 out]
        n206 = global write "GR_Servo.vi" "Error Message"(w360) -> ()
      }
    }
    n207 = global read "Galobal variable_TI.vi" "Auto Exit"() -> (w65:bool)
  }
  n208 = local write "Error   For Message"(w4) -> ()
  n209 = global write "Galobal variable_TI.vi" "Errror For Color"(w4) -> ()
  n210 = local write "Start"(T7 FALSE ("Start")) -> ()
  n211 = Get Date/Time In Seconds() -> (seconds since 1Jan1904=w34:timestamp)
  n212 = while {
    shift-right: [w438] -> _
    shift-left: w34 -> [w437]
    tunnel: w4 -> [_]
    stop <- w435 stop-if-true
    n213 = global read "Galobal variable_TI.vi" "Sensor Setting Data"() -> (w413:T15)
    n214 = global read "Galobal variable_TI.vi" "Camera OK"() -> (w420:bool)
    "Camera" <- w420
    n215 = global read "Galobal variable_TI.vi" "Sensor Data"() -> (w414:T16)
    n216 = global read "Galobal variable_TI.vi" "Camera NG"() -> (w419:bool)
    "Camera" <- w419
    n217 = global read "Galobal variable_TI.vi" "NI Comm.Error"() -> (→"Error":bool)
    n218 = global read "Galobal variable_TI.vi" "Errror For Color"() -> (w415:bool)
    n219 = Get Date/Time In Seconds() -> (seconds since 1Jan1904=w434:timestamp)
    "Current Date & Time" <- w434
    n220 = local read "Error   For Message"() -> (w400:bool)
    n221 = Unbundle By Name(w414) -> ("IL Sensor1_AI0"=w411:dbl, "IL Sensor1_AI1"=w410:dbl, "IL Sensor1_AI0"=w409:bool, "IL Sensor1_AI1"=w408:bool)
    n222 = Unbundle By Name(w413) -> ("IL Sensor1_Max AI0"=w406:dbl, "IL Sensor1_Min AI0"=w405:dbl, "IL Sensor1_Max AI1"=w404:dbl, "IL Sensor1_ Min AI1"=w403:dbl)
    n223 = global write "Galobal variable_TI.vi" "Stop M1"("Stop") -> ()
    n224 = property on="Camera" class="Bool (strict)"("Visible"=w420) -> ()  [unwired: 2 in, 2 out]
    n225 = case shown="False" "Cycle Start Bit" {
      tunnel: w437 -> [_ w441]
      tunnel: w434 -> [w439 w442]
      tunnel: [w439 w441] -> w438
      frame False {
      }
      frame True {
        n226 = Subtract(x=w442, y=w441) -> (x-y=w443:dbl)
        n227 = To Long Integer(number=w443) -> (32bit integer=w440:i32)
        "Cycle Time(Sec)" <- w440
        n228 = local write "Cycle"(w440) -> ()
      }
    }
    n229 = property on="Camera" class="Bool (strict)"("Visible"=w419) -> ()  [unwired: 2 in, 2 out]
    n230 = Bundle By Name(cluster=T2 {"Keypad_AI0"=0.07252740645964428, "Keypad_AI1"=5.026581771182417, "Keypad_AI0"=FALSE, "Keypad_AI1"=TRUE} ("Sensor Data 2"), "Keypad_AI0"=w411, "Keypad_AI1"=w410, "Keypad_AI0"=w409, "Keypad_AI1"=w408) -> (→"Sensor Data":T2)
    n231 = global read "Galobal variable_TI.vi" "Cordinate"() -> (→"Co-ordinate":string)
    n232 = Select(t=enum32{"Test", "Report"}."Report" ("Tab Control"), s="Report", f=enum32{"Test", "Report"}."Test" ("Tab Control")) -> (s? t:f=w423:enum32{"Test", "Report"})
    n233 = Or(x=w415, y=w400) -> (x .or. y?=w401:bool)
    n234 = global read "Galobal variable_TI.vi" "Auto Exit"() -> (w435:bool)
    n235 = Get Date/Time In Seconds() -> (seconds since 1Jan1904=w430:timestamp)
    n236 = global read "Galobal variable_TI.vi" "Running Model"() -> (→"Running Model":string)
    n237 = global read "Galobal variable_TI.vi" "LCD Barcode"() -> (→"TFT Barcode":string)
    n238 = global read "Galobal variable_TI.vi" "MIC Barcode"() -> (→"MIC Barcode":string)
    n239 = local write "Tab Control"(w423) -> ()
    n240 = Bundle By Name(cluster=T1 {"Keypad_Max AI0"=58.0, "Keypad_Min AI0"=3.0, "Keypad_Max AI1"=5.4, "Keypad_ Min AI1"=3.0} ("Sensor Setting Data 2"), "Keypad_Max AI0"=w406, "Keypad_Min AI0"=w405, "Keypad_Max AI1"=w404, "Keypad_ Min AI1"=w403) -> (→"Sensor Setting Data":T1)
    n241 = Select(t=u32 16711680, s=w401, f=u32 16777226) -> (s? t:f=w418:u32)
    n242 = global read "Galobal variable_TI.vi" "Server"() -> (→"Boolean 2":bool)
    n243 = Format Date/Time String(time format string (%c)="%d-%m-%Y  %H:%M:%S", seconds (now)=w430) -> (date/time string=→"Date time":string)  [unwired: 1 in]
    n244 = property on="Error Message" class="Str"("Text.BGColor"=w418) -> ()  [unwired: 2 in, 2 out]
  }
  n245 = while {
    stop <- w445 stop-if-true
    n246 = event shown="[0] Timeout" {
      selector: _ -> [_ _ _]
      dyn-events: _ -> [_ _ _]
      timeout: 100 -> [_ _ _]
      event Timeout {
        n247 = event-data() -> ()  [unwired: 1 in, 3 out]
        n248 = global read "GR_Servo.vi" "Error Message"() -> (→"Error Message":string)
        n249 = global read "Galobal variable_TI.vi" "Digital input"() -> (w472:bool[])
        n250 = global read "Galobal variable_TI.vi" "Digital input"() -> (w481:bool[])
        n251 = Index Array(array=w472, index #1=25 ("index"), index #2=26 ("index"), index #3=27 ("index"), index #4=28 ("index"), index #5=16 ("index"), index #6=17 ("index"), index #7=18 ("index")) -> (element #1=→"Cllip-1 (AI9)":bool, element #2=→"Cllip-2(AI10)":bool, element #3=→"Cllip-4 (AI12)":bool, element #4=→"Cllip-3 (AI11)":bool, element #5=→"Key Pad AI0":bool, element #6=→"Key Pad AI1":bool, element #7=w459:bool)
        n252 = Not(x=w459) -> (.not. x?=→"Servo Fault":bool)
        n253 = Index Array(array=w481, index #1=0 ("index"), index #2=8 ("index"), index #3=2 ("index")) -> (element #1=→"Start":bool, element #2=w477:bool, element #3=→"reset":bool)
        n254 = global read "Galobal variable_TI.vi" "Digital input"() -> (w455:bool[])
        n255 = global read "Galobal variable_TI.vi" "STM Done Bit"() -> (w478:bool)
        n256 = Or(x=w477, y=w478) -> (x .or. y?=w476:bool)
        n257 = Index Array(array=w455, index #1=0 ("index"), index #2=1 ("index"), index #3=2 ("index"), index #4=3 ("index")) -> (element #1=→"Start":bool, element #2=w449:bool, element #3=→"Reset":bool, element #4=→"Home":bool)
        n258 = Select(t=cluster{u32, u32}[] [{16734762, 6618880}, {16777222, 6618880}] ("Colors [4]"), s=w476, f=cluster{u32, u32}[] [{16734762, 16711680}, {16777222, 16775560}] ("Colors [4]")) -> (s? t:f=w482:cluster{u32, u32}[])
        n259 = Not(x=w449) -> (.not. x?=→"Emergency":bool)
        n260 = property on="Slide Servo Home Call" class="Bool (strict)"("Colors [4]"=w482) -> ()  [unwired: 2 in, 2 out]
      }
      event "Servo Fault Reset": Value Change {
        n261 = event-data() -> ("NewVal"=w485:bool)  [unwired: 1 in]
        n262 = global read "Galobal variable_TI.vi" "Manual DO"() -> (w488:bool[])
        n263 = Replace Array Subset(array=w488, new element=w485, index=1) -> (w487:bool[])
        n264 = global write "Galobal variable_TI.vi" "Manual DO"(w487) -> ()
      }
      event Value Change {
        n265 = event-data() -> ("NewVal"=w489:T8)  [unwired: 1 in]
        n266 = global write "Galobal variable_TI.vi" "Auto Exit"(w489) -> ()
      }
    }
    n267 = local read "Exit"() -> (w445:T8)
  }
  n268 = call "Auotmode.vi"("Enum Selection"=Auot_Test_selection."Flush", "Error In"=w29, "queue in"=w35) -> ("error out"=w40:errorcluster, "queue Out"=w39:refnum<queue>)  [unwired: 5 in, 1 out]
  n269 = call "Auotmode.vi"("Enum Selection"=Auot_Test_selection."Release Queue", "Error In"=w40, "queue in"=w39) -> ("error out"=→"error out":errorcluster)  [unwired: 5 in, 2 out]
